vi "measure.vi"(11 "Qube":refnum<class "Qube.lvclass">) -> (0 "y":dbl[](array[numeric]), 3 "Qube":refnum<class "Qube.lvclass">, 4 "counts":i32)   [LabVIEW 2020, in "Qube.lvclass"]
uses:
  Qube.lvclass
  Qube.lvclass/Qube.ctl
  <vilib>/Quanser/Rapid Control Prototyping Toolkit/hardware/HIL Board/HIL Read.vi
  <vilib>/Quanser/Rapid Control Prototyping Toolkit/hardware/HIL Board/_TypeSpecific/HIL Read Encoder (Scalar).vi
  <vilib>/Quanser/Rapid Control Prototyping Toolkit/hardware/HIL Board/HIL Board.lvclass
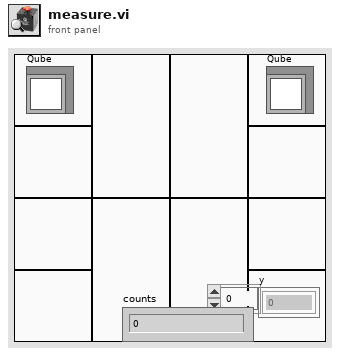
[diagram p1: front panel]
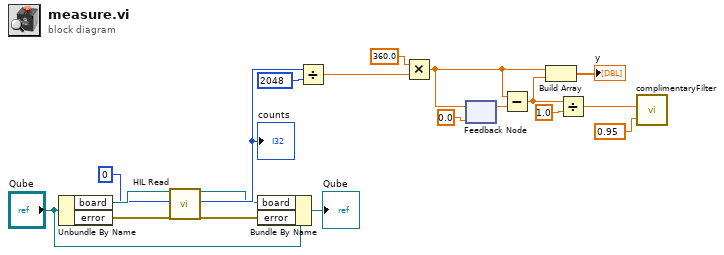
[diagram p0: block diagram]
diagram:
  n1 = Unbundle By Name("Qube") -> ("board"=w18:refnum<class "HIL Board.lvclass">, "error"=w19:errorcluster)
  n2 = call-poly "HIL Read"("board in"=w18, "channel"=u32 0, "error in (no error)"=w19) -> ("board out"=w6:refnum<class "HIL Board.lvclass">, "counts"=w17:i32, "error out"=w13:errorcluster)  [unwired: 14 in]
  "counts" <- w17
  n3 = Bundle By Name(cluster="Qube", "board"=w6, "error"=w13) -> (→"Qube":refnum<class "Qube.lvclass">)
  n4 = Divide(x=w17, y=2048) -> (x/y=w15:dbl)
  n5 = Multiply(x=360.0, y=w15) -> (x*y=w2:dbl)
  n6 = feedback-in #1(w2) -> ()
  n7 = feedback #1(0.0) -> (w8:dbl)
  n8 = Subtract(x=w2, y=w8) -> (x-y=w1:dbl)
  n9 = Build Array(w2, w1) -> (→"y":dbl[])
  n10 = Divide(x=w1, y=1.0) -> (x/y=w4:dbl)
  n11 = call "complimentaryFilter.vi"("alpha"=0.95, "low pass component"=w4) -> ()  [unwired: 9 in, 1 out]
